vi "Write wildcard.vi"(8 "error in (no error)":errorcluster, 10 "prefix":string, 11 "wildcards in":refnum<class "wildcards.lvclass">) -> (0 "error out":errorcluster, 3 "wildcards out":refnum<class "wildcards.lvclass">)   [LabVIEW 2023, in "uLib.lvlib" / "wildcards.lvclass"]
uses:
  wildcards.lvclass
  wildcards.lvclass/wildcards.ctl
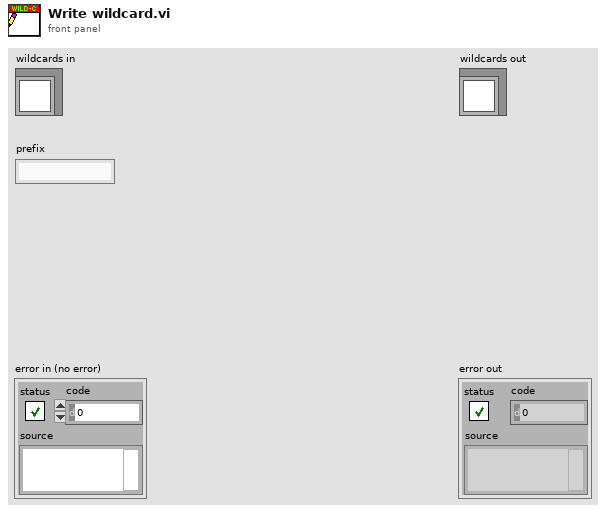
[diagram p1: front panel]
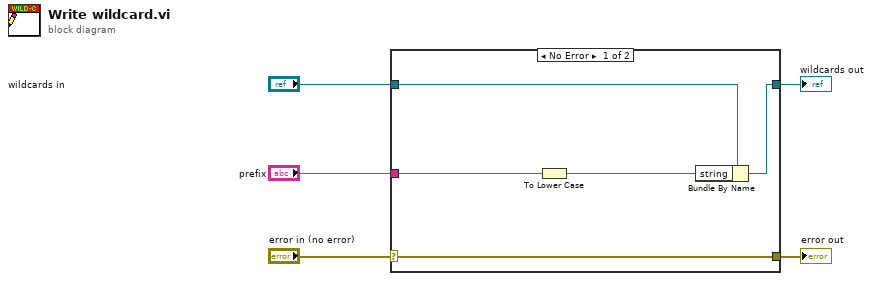
[diagram p0: block diagram]
diagram:
  n1 = case shown="No Error" "error in (no error)" {
    selector: "error in (no error)" -> [w10 w11]
    tunnel: [w10 w11] -> w4
    tunnel: [w8 w12] -> w2
    tunnel: "wildcards in" -> [w9 w12]
    tunnel: "prefix" -> [w7 _]
    frame No Error {
      n2 = To Lower Case(string=w7) -> (all lower case string=w6:string)
      n3 = Bundle By Name(cluster=w9, "string"=w6) -> (w8:refnum<class "wildcards.lvclass">)
    }
    frame Error {
    }
  }
  "error out" <- w4
  "wildcards out" <- w2
